vi "S2C_FORNAX_Poly_SystemConfigurationCommand.vi"(8 "Error In":errorcluster, 10 "SystemConfigurationCommand":T2={"Partition"="Default", "Message"="SystemConfigurationCommand", "M_Command"=0, "M_ConfigurationData"=""} {"M_Command" items=["SYSTEM_CONFIG_CMD_NONE", "SYSTEM_CONFIG_CMD_READ_CONFIG", "SYSTEM_CONFIG_CMD_WRITE_CONFIG", "SYSTEM_CONFIG_CMD_SW_UPDATE_ENTER", "SYSTEM_CONFIG_CMD_SW_UPDATE_START", "SYSTEM_CONFIG_CMD_SW_UPDATE_EXIT", "SYSTEM_CONFIG_CMD_UPDATE_ONE_BOARD_CHASSIS_INFO", "SYSTEM_CONFIG_CMD_UPDATE_ALL_BOARDS_CHASSIS_INFO", "SYSTEM_CONFIG_CMD_READ_ONE_BOARD_INFO", "SYSTEM_CONFIG_CMD_READ_ALL_BOARDS_INFO", "SYSTEM_CONFIG_CMD_REGISTER_BOARD", "SYSTEM_CONFIG_CMD_APPROVE_CURRENT_CONFIG", "SYSTEM_CONFIG_CMD_ROTATE_EVENT_LOGS", "SYSTEM_CONFIG_CMD_SYSTEM_RESTART", "SYSTEM_CONFIG_CMD_ROTATE_USAGE_LOGS", "SYSTEM_CONFIG_CMD_ENTER_SERVICE", "SYSTEM_CONFIG_CMD_EXIT_SERVICE", "SYSTEM_CONFIG_CMD_SW_UPDATE_CONFIRM", "SYSTEM_CONFIG_CMD_ROTATE_ALL_LOGS"]}, 11 "Settings":T3={"Driver"="Fornax", "Command"="SystemConfigurationCommand", "Return"="ErrorStatus", "Parameters"="", "Timeout"=10.0}) -> (0 "Error Out":errorcluster, 3 "Response":string)   [LabVIEW 2015]
uses:
  Typedefs/SystemConfigurationCommand.ctl
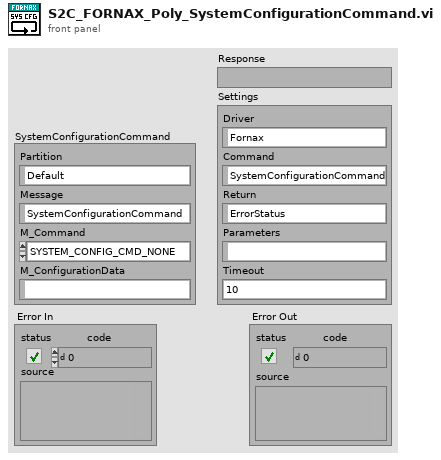
[diagram p1: front panel]
types:
  T1 = typedef "SystemConfigurationCommand.ctl" = i16
  T2 = cluster{"Partition":string, "Message":string, "M_Command":T1, "M_ConfigurationData":string}
  T3 = cluster{"Driver":string, "Command":string, "Return":string, "Parameters":string, "Timeout":dbl}
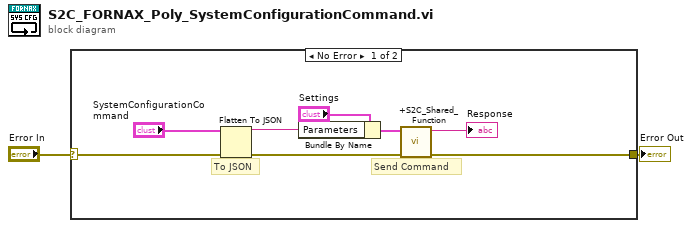
[diagram p0: block diagram]
diagram:
  n1 = case shown="No Error" "Error In" {
    selector: "Error In" -> [w6 w11]
    tunnel: [w5 w11] -> w1
    frame No Error {
      # "To JSON"
      # "Send Command"
      n2 = Flatten To JSON(anything="SystemConfigurationCommand", error in (no error)=w6) -> (JSON string=w7:string, 11:w9:errorcluster)  [unwired: 1 in]
      n3 = Bundle By Name(cluster="Settings", "Parameters"=w7) -> (w10:T3)
      n4 = call "+S2C_Shared_Function.vi"("Error In"=w9, "Settings"=w10) -> ("Error Out"=w5:errorcluster, "Response"=→"Response":string)  [unwired: 8 in]
    }
    frame Error {
    }
  }
  "Error Out" <- w1
